vi "SameGroup.vi"(8 "error in (no error)":errorcluster, 10 "SelectionType":refnum<class "MGI_SelectionType.lvclass">, 11 "RadioSelection in":refnum<class "MGI_RadioSelection.lvclass">) -> (0 "error out":errorcluster, 2 "Same Group?":bool, 3 "RadioSelection out":refnum<class "MGI_RadioSelection.lvclass">)   [LabVIEW 2016, in "MGI_RadioSelection.lvclass"]
doc: "Determines if the two items are in the same radio group.\n\nAuthored by Derek E. Trepanier\nsupport@mooregoodideas.com\nwww.mooregoodideas.com\n\nCopyright (c) 2012, Moore Good Ideas, Inc.\n\nAll rights reserved.\n\nRedistribution and use in source and binary forms, with or without modification, are permitted provided that the following conditions are met:\n\n * Redistributions of source code must retain the above copyright notice, this list of conditions and the following disclaimer.\n * Redistributions in binary form must reproduce the above copyright notice, this list of conditions and the following disclaimer in the documentation and/or other materials provided with the distribution.\n * Neither the name of Moore Good Ideas, Inc. nor the names of its contributors may be used to endorse or promote products derived from this software without specific prior written permission.\n\nTHIS SOFTWARE IS PROVIDED BY THE COPYRIGHT HOLDERS AND CONTRIBUTORS \"AS IS\" AND ANY EXPRESS OR IMPLIED WARRANTIES, INCLUDING, BUT NOT LIMITED TO, THE IMPLIED WARRANTIES OF MERCHANTABILITY AND FITNESS FOR A PARTICULAR PURPOSE ARE DISCLAIMED. IN NO EVENT SHALL THE COPYRIGHT OWNER OR CONTRIBUTORS BE LIABLE FOR ANY DIRECT, INDIRECT, INCIDENTAL, SPECIAL, EXEMPLARY, OR CONSEQUENTIAL DAMAGES (INCLUDING, BUT NOT LIMITED TO, PROCUREMENT OF SUBSTITUTE GOODS OR SERVICES; LOSS OF USE, DATA, OR PROFITS; OR BUSINESS INTERRUPTION) HOWEVER CAUSED AND ON ANY THEORY OF LIABILITY, WHETHER IN CONTRACT, STRICT LIABILITY, OR TORT (INCLUDING NEGLIGENCE OR OTHERWISE) ARISING IN ANY WAY OUT OF THE USE OF THIS SOFTWARE, EVEN IF ADVISED OF THE POSSIBILITY OF SUCH DAMAGE."
uses:
  <userlib>/_MGI/Menu Building/SelectionType/RadioSelection/MGI_RadioSelection.lvclass
  <userlib>/_MGI/Menu Building/SelectionType/MGI_SelectionType.lvclass
  <userlib>/_MGI/Menu Building/SelectionType/RadioSelection/MGI_RadioSelection.lvclass/MGI_RadioSelection.ctl
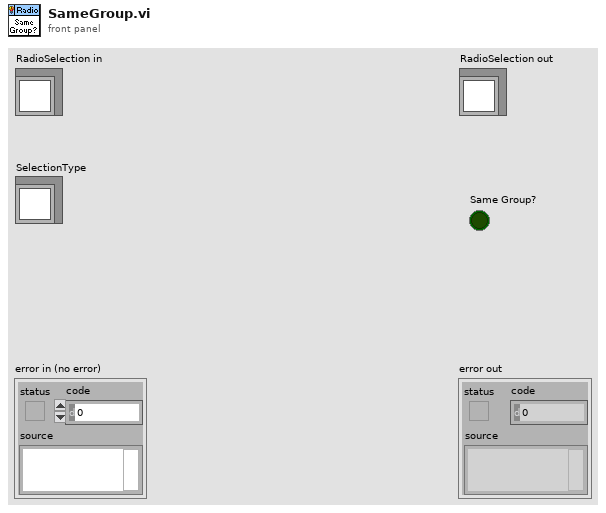
[diagram p1: front panel]
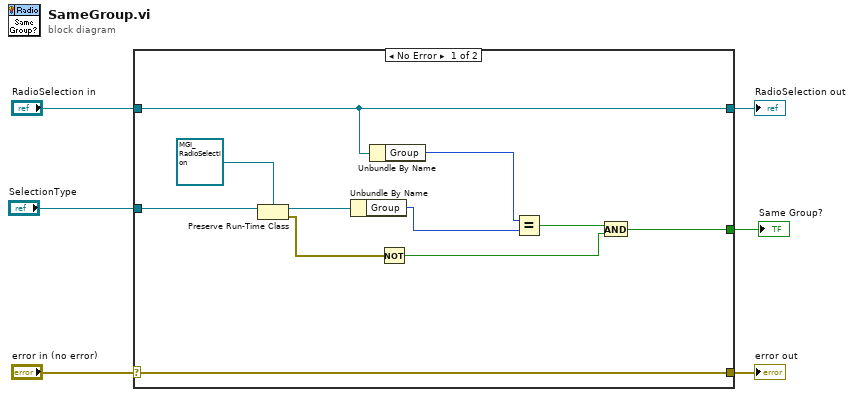
[diagram p0: block diagram]
diagram:
  n1 = case shown="No Error" "error in (no error)" {
    selector: "error in (no error)" -> [w17 w19]
    tunnel: [w17 w19] -> w5
    tunnel: [w10 w18] -> w3
    tunnel: "RadioSelection in" -> [w10 w18]
    tunnel: "SelectionType" -> [w16 _]
    tunnel: [w12 _] -> w1
    frame No Error {
      n2 = Preserve Run-Time Class(object in=w16, 2:refnum<class "MGI_RadioSelection.lvclass"> refnum ("RadioSelection.lvclass")) -> (object out=w8:refnum<class "MGI_RadioSelection.lvclass">, error out=w14:errorcluster)  [unwired: 1 in]
      n3 = Unbundle By Name(w8) -> ("Group"=w7:u8)
      n4 = Unbundle By Name(w10) -> ("Group"=w9:u8)
      n5 = Not(x=w14) -> (.not. x?=w13:bool)
      n6 = Equal?(x=w9, y=w7) -> (x = y?=w15:bool)
      n7 = And(x=w15, y=w13) -> (x .and. y?=w12:bool)
    }
    frame Error {
    }
  }
  "error out" <- w5
  "RadioSelection out" <- w3
  "Same Group?" <- w1
